vi "Parser.vi"(8 "error in (no error)":errorcluster, 10 "RIO device address":string="rio://GEcoPharLap18sp1/RIO0", 11 "bitfile path":path=path "C:/Users/nitest/Desktop/Mockup/FPGA Bitfiles/Project_FPGATarget_FPGAVI_CScS9XDPUnU.lvbitx") -> (0 "error out":errorcluster, 2 "FXP channels out":T1(array[cluster]), 3 "session out":u64)   [LabVIEW 2018]
uses:
  D:/GitBranches/niveristand-fpga-addon-custom-device-1/Source/Addon/Addon System Explorer/FPGA Addon System Explorer.lvlib
  NiFpga.dll
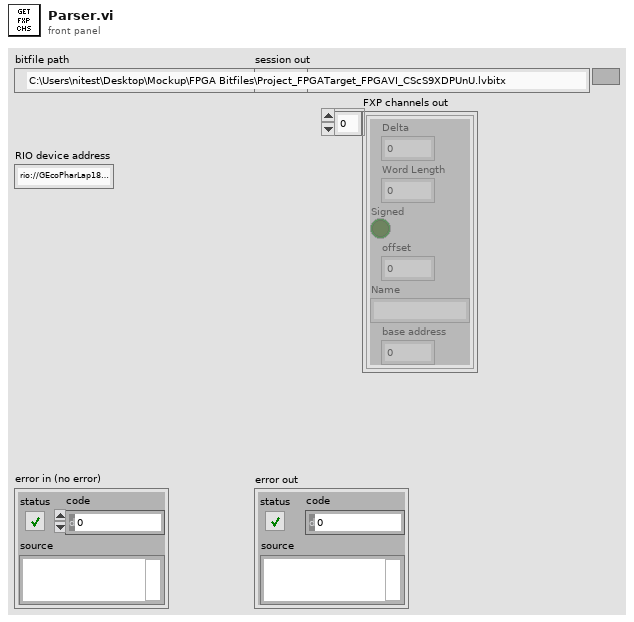
[diagram p1: front panel]
types:
  T1 = cluster{"Delta":dbl, "Word Length":i8, "Signed":bool, "offset":i32, "Name":string, "base address":i32}[]
  T2 = typedef "niFpgaBitfileStructure_VI.ctl" = cluster{"Name":string, "RegisterMap":T3[], "Icon":T8}
  T3 = typedef "nirviControlStructure.ctl" = cluster{"Name":string, "Hidden":bool, "Indicator":bool, "Flattened Type":string, "Grouping":cluster{"Grouped":bool, "Member Names":string[], "Member IDs":u32[]}, "Address":u32, "Size":u32, "Class":u32, "Internal":bool, "Typedef":T4, "ID":u32, "Bidirectional":bool, "Synchronous":bool, "Mechanical Action":T5, "Sub Controls":T6[], "Access May Timeout":bool, "Register Node":bool}
  T4 = typedef "nirviTypdefDescription.ctl" = cluster{"Typedef":bool, "Path":path}
  T5 = typedef "nirviMechanicalAction.ctl" = enum8{"Switch When Pressed", "Switch When Released", "Switch Until Released", "Latch When Pressed", "Latch When Released", "Latch Until Released"}
  T6 = typedef "nirviSubControlStructure.ctl" = cluster{"Name":string, "flattened Type":string, "Cluster Information":T7, "Typedef":T4}
  T7 = typedef "nirviClusterElementControl.ctl" = cluster{"Name Hierarchy":string[], "Item Order":u32[]}
  T8 = typedef "imagedata.ctl" = cluster{"image type":i32, "image depth":i32, "image":u8[], "mask":u8[], "colors":u32[], "Rectangle":cluster{"left":i16, "top":i16, "right":i16, "bottom":i16}}
  T9 = cluster{"Delta":dbl, "Word Length":i8, "Signed":bool, "offset":i32, "Name":string, "base address":i32}
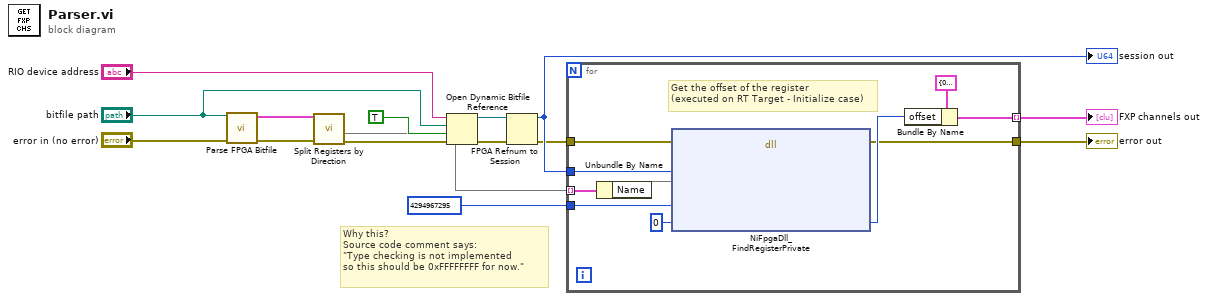
[diagram p0: block diagram]
diagram:
  # "Why this?\nSource code comment says:\n\"Type checking is not implemented \nso this should be 0xFFFFFFFF for now.\""
  n1 = call "Parse FPGA Bitfile.vi"("error in (no error)"="error in (no error)", "Path"="bitfile path") -> ("error out"=w15:errorcluster, "vi info"=w14:T2)  [unwired: 7 in, 1 out]
  n2 = call "Split Registers by Direction.vi"("error in"=w15, "vi info"=w14) -> ("error out"=w13:errorcluster, 1:w2)  [unwired: 6 in, 2 out]
  n3 = Open Dynamic Bitfile Reference(0:"RIO device address", 1:"bitfile path", 2:TRUE ("Run When Loaded"), 3:w13) -> (5:w8:refnum<k20>, 8:w9:errorcluster)  [unwired: 1 in]
  n4 = FPGA Refnum to Session(4:w9, 7:w8) -> (0:w6:errorcluster, 3:w7:u64)
  "session out" <- w7
  n5 = for {
    tunnel: w7 -> [w25]
    tunnel: w6 -> [w24]
    tunnel: u32 4294967295 -> [w22]
    tunnel: [w20] -> w3
    tunnel: w2 -> [w19] mode=indexing
    tunnel: [w16] -> w1 mode=indexing
    # "Get the offset of the register\n(executed on RT Target - Initialize case)"
    n6 = Unbundle By Name(w19) -> ("Name"=w18)
    n7 = dll-call lib="NiFpga.*" fn="NiFpgaDll_FindRegisterPrivate"(error in=w24, "session"=w25, "registerName"=w18, "expectedResourceType"=w22, "resourceOffset"=u32 0) -> (error out=w20:errorcluster, "resourceOffset"=w21:u32)  [unwired: 6 in, 1 out]
    n8 = Bundle By Name(cluster=T9 {"Delta"=0.0, "Word Length"=0, "Signed"=FALSE, "offset"=0, "Name"="", "base address"=0}, "offset"=w21) -> (w16:T9)
  }
  "error out" <- w3
  "FXP channels out" <- w1
